vi "Parse State Queue++.vi"(0 "State Queue":string, 1 "Name(\"\" to use uuid)":string, 7 "Error In (no error)":errorcluster, 9 "Dequeue Timeout(0ms)":i32, 11 "Response Timeout(1000ms)":i32=10000) -> (4 "Remaining States":string, 6 "Current State":string, 8 "Arguments":string, 15 "From Who":string)   [LabVIEW 2014, in "JKI-State-Machine-Plus.lvlib"]
doc: "Parses the JKI State Machine state queue and returns the current state that will execute next with the associated arguments.\n\nFor instructions on how to use the JKI State Machine, examples and video tutorials, visit:\nhttp://jkisoft.com/state-machine/\n\n<B>Inputs:</B>\n <B>State Queue:</B> The entire state queue is wired to this input. This should come from the main JKI State Machine shift register.\n <B>Error In</B> The error cluster from the JKI State Machine is wired to this input. If an error occures and appears on this input, the current state output returns the \"Error Handler\" state.\n\n<B>Outputs:</B>\n <B>Remaining States:</B> Returns all the next states that should execute after the current state completes. These should be passed through the current state in the state machine. These can also be modified or augmented within the current state if necessary.\n <B>Current State:</B> Returns the current state that should execute next in the state machine. If an error is wired to the Error input then the current state output becomes \"Error Handler\".\n <B>Arguments:</B> Returns any argument(s) that may be used in the current state string. These arguments come after the \">>\" characters. <B>Note:</B> The arguments variable must not contain any unprintable characters like linefeed or carriage return.\n\n<B>State Syntax:</B>\nStateCategory: State >> Argument\nLine Terminator: Line feed\n <B>Example:</B>\nUI: Help >> About\n\nWhere \"UI\" is the state category\nWhere \"Help\" is the state\nWhere \"About\" is the argument\n <B>Other Examples:</B>\nApp Data: Initialize\nUI: Initialize\nHelp >> About\n\n<B>Commenting:</B>\nTo add a comment use \"//\" or \"#\" and all text to the right will be ignored\n <B>Commenting Example:</B>\nUI: Initialize // This initializes the UI\n# This whole line is a comment\n// Another comment line\n\nJKI State Machine™ 2018.0.7.45\nhttp://jki.net/state-machine/\nCopyright (C) 2005-2018, JKI <info@jki.net>\nALL RIGHTS RESERVED"
uses:
  JKI-State-Machine-Plus.lvlib
  _Support/_Cross JKI StateMachine State Data.ctl
  _Support/_Cross JKI StateMachine State Response.ctl
  _Support/_uuid.vi
  <vilib>/addons/_JKI Toolkits/State Machine/_JKI_lib_State_Machine.llb/Add State(s) to Queue__JKI_lib_State_Machine.vi
  Build State String with Arguments++.vi
  _Support/_JKISMQFGV.vi
  <vilib>/regexp/Match Regular Expression.xnode
panel:
  # "For instructions on how to use the JKI State Machine, examples and video tutorials, visit:\nhttp://jki.net/state-machine/\n\nJKI State Machine™\nhttp://jki.net/state-machine/\nCopyright (C) 2005-2017, JKI <info@jki.net>\nALL RIGHTS RESERVED"
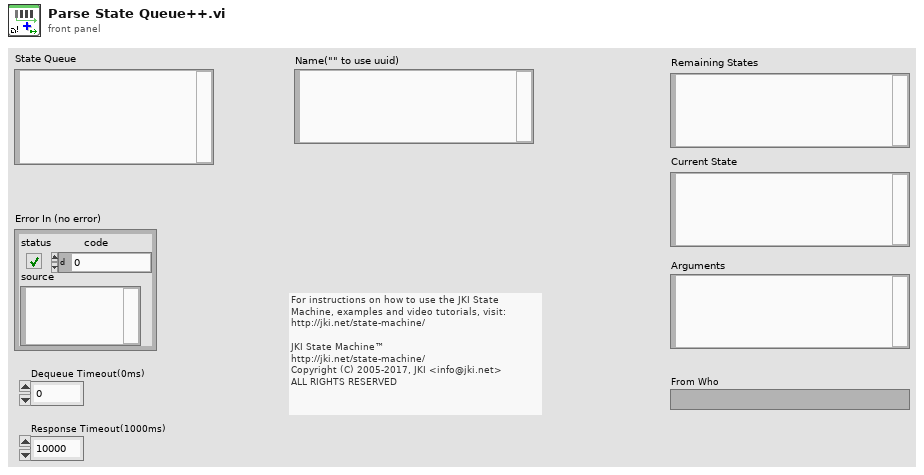
[diagram p1: front panel]
types:
  T1 = typedef "JKI-State-Machine-Plus.lvlib/_Cross JKI StateMachine State Data.ctl" = cluster{"state":string, "args":string, "source":string, "RespQ":refnum<queue>}
  T2 = typedef "JKI-State-Machine-Plus.lvlib/_Cross JKI StateMachine State Response.ctl" = cluster{"error":errorcluster}
  T3 = typedef "JKI-State-Machine-Plus.lvlib/_JKISMQ.ctl" = cluster{"Queue":refnum<queue>, "Locked Status":refnum<data-value>, "Stand Alone Mode":bool}
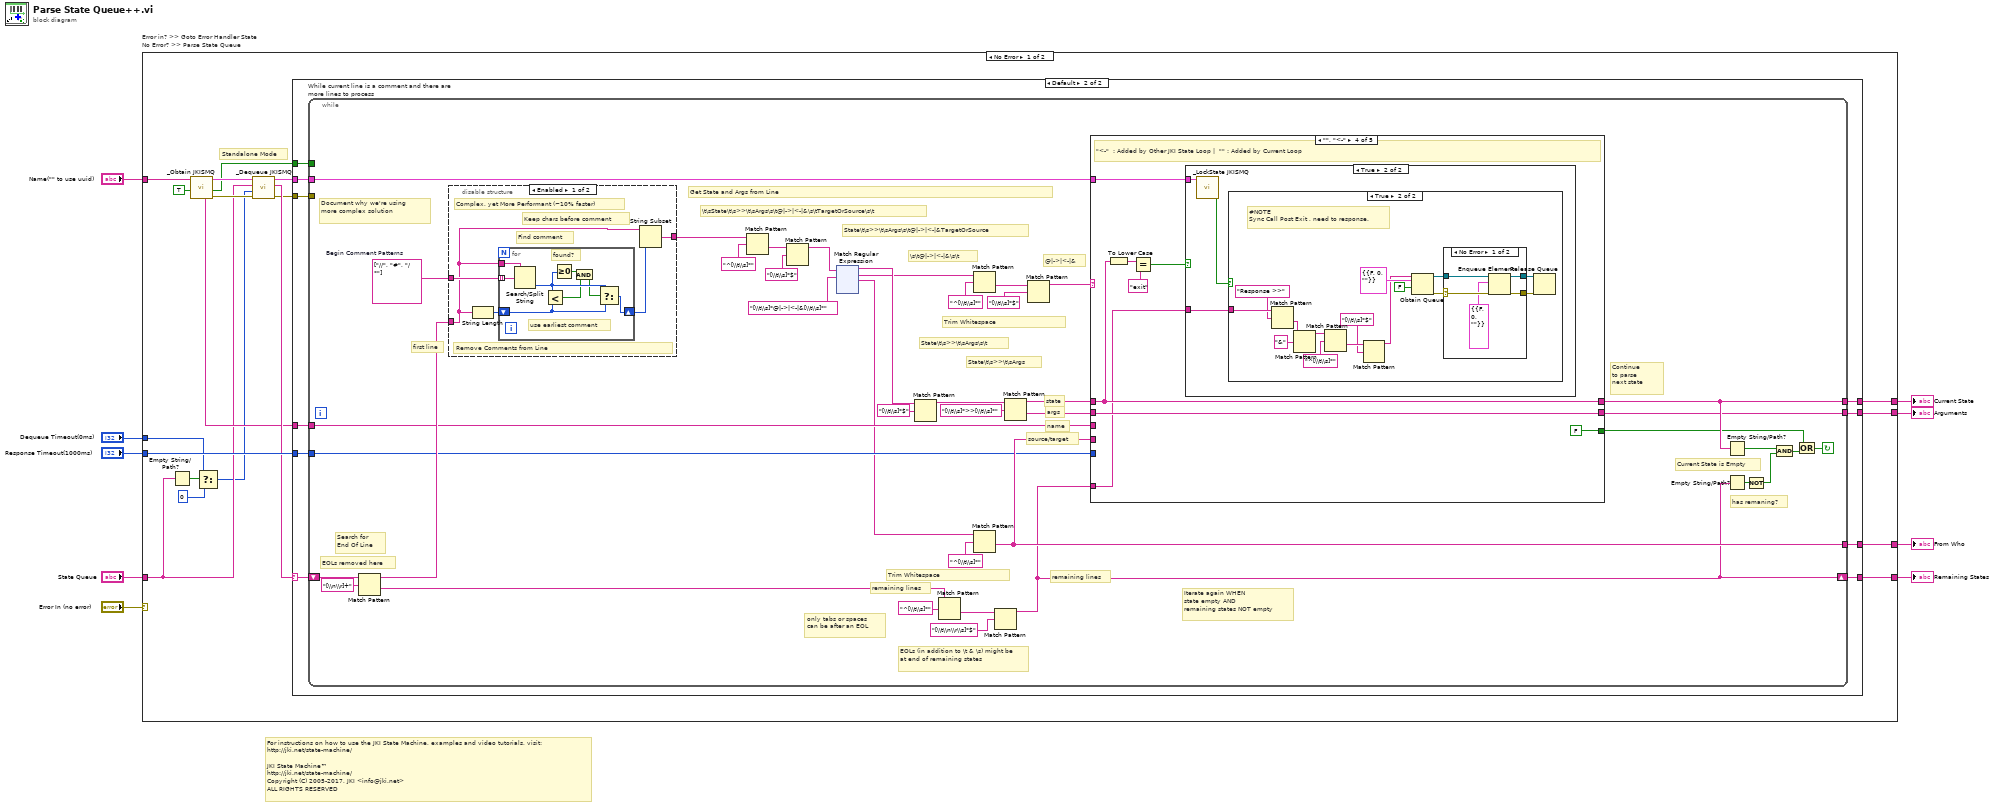
[diagram p0: block diagram]
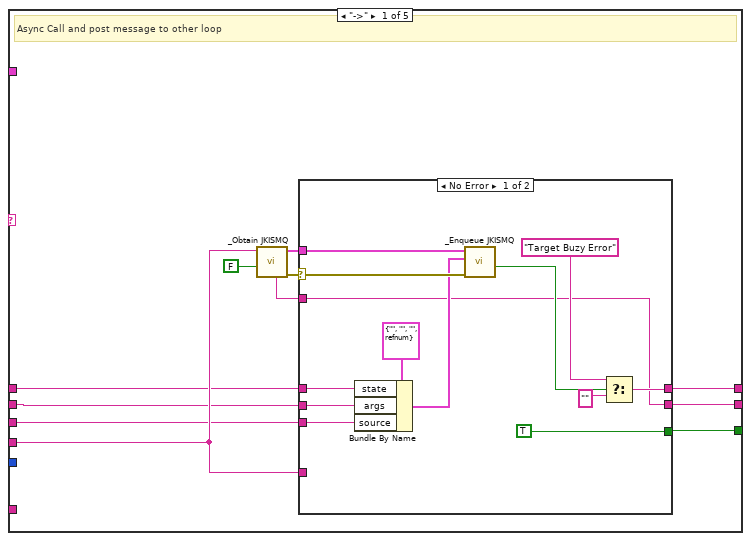
[diagram p3: hidden frame]
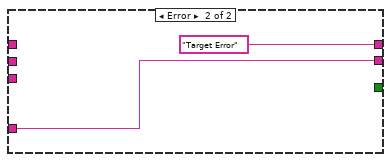
[diagram p4: hidden frame]
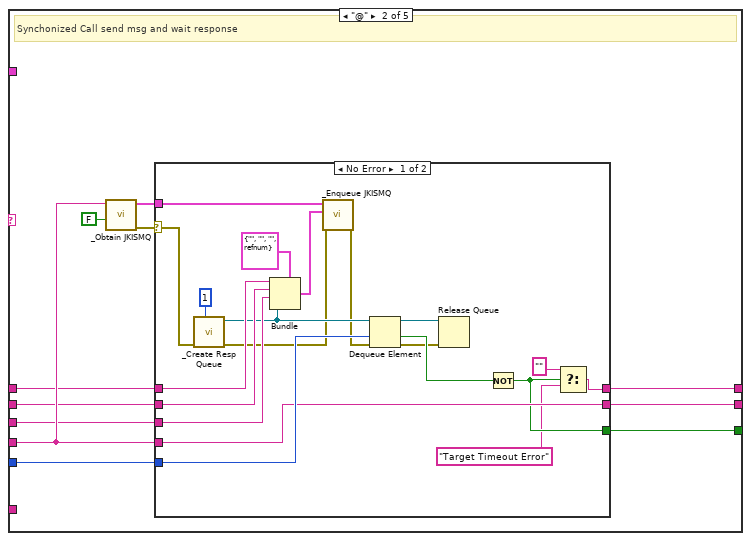
[diagram p5: hidden frame]
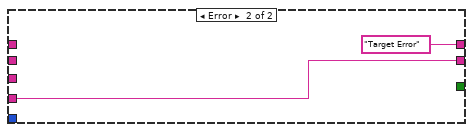
[diagram p6: hidden frame]
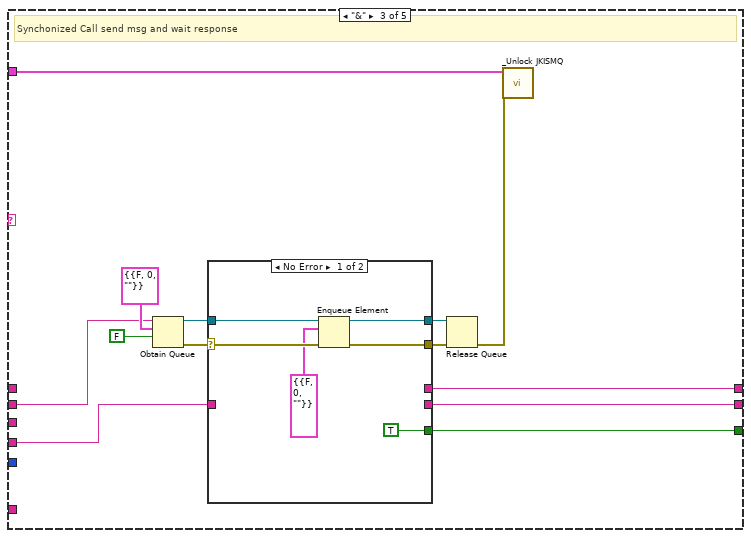
[diagram p7: hidden frame]
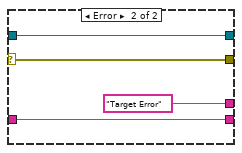
[diagram p8: hidden frame]
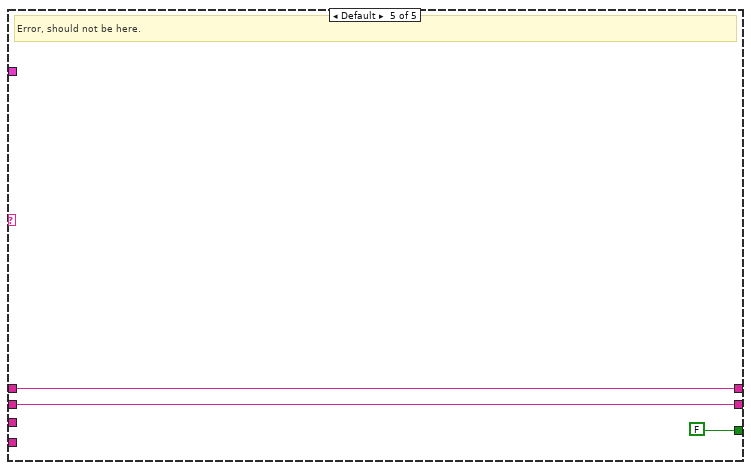
[diagram p12: hidden frame]
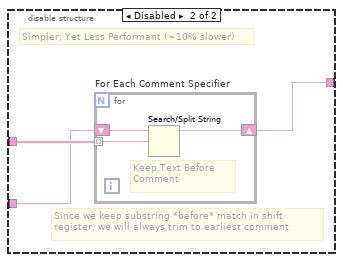
[diagram p13: hidden frame]
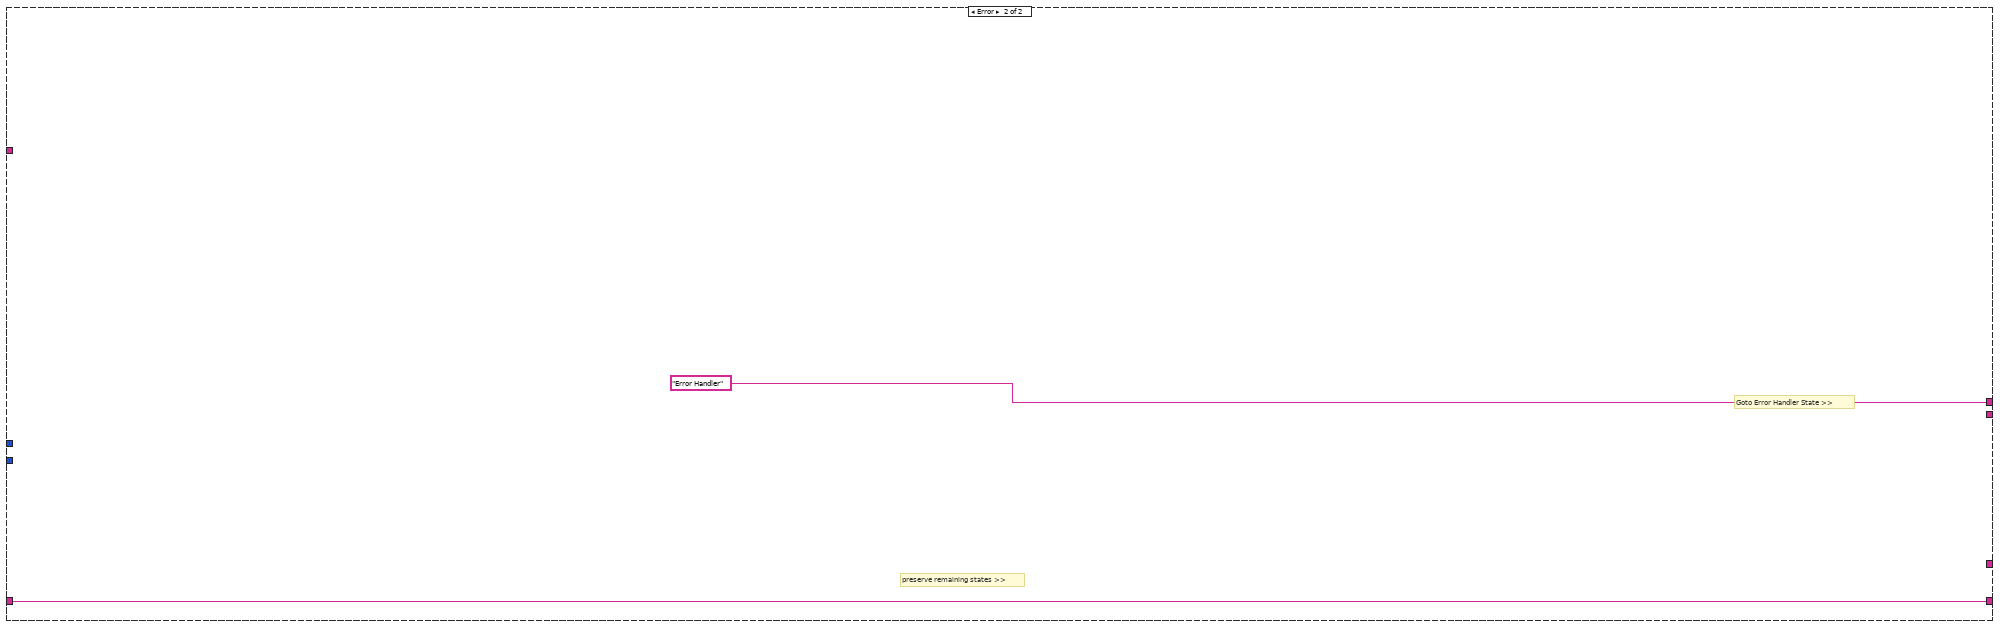
[diagram p14: hidden frame]
diagram:
  # "For instructions on how to use the JKI State Machine, examples and video tutorials, visit:\nhttp://jki.net/state-machine/\n\nJKI State Machine™\nhttp://jki.net/state-machine/\nCopyright (C) 2005-2017, JKI <info@jki.net>\nALL RIGHTS RESERVED"
  n1 = case "Error in? >> Goto Error Handler State\nNo Error? >> Parse State Queue" shown="No Error" "Error In (no error)" {
    tunnel: [w26 w331] -> w9
    tunnel: [w28 "Error Handler"] -> w7
    tunnel: [w27 _] -> w6
    tunnel: "State Queue" -> [w14 w331]
    tunnel: "Response Timeout(1000ms)" -> [w25 _]
    tunnel: "Name(\"\" to use uuid)" -> [w24 _]
    tunnel: [w23 _] -> w2
    tunnel: "Dequeue Timeout(0ms)" -> [w13 _]
    frame No Error {
      # "Standalone Mode"
      n2 = Empty String/Path?(string/path=w14) -> (empty?=w15:bool)
      n3 = call "_Obtain JKISMQ.vi"("create if not found? (T)"=TRUE, "Name(\"\" to use uuid) in"=w24) -> ("Error out"=w20:errorcluster, "Stand Alone Mode"=w10:bool, "JKISMQ"=w22:T3, "Name"=w17:string)  [unwired: 6 in]
      n4 = Select(t=w13, s=w15, f=0) -> (s? t:f=w11:i32)
      n5 = call "_Dequeue JKISMQ.vi"("Error in"=w20, "Dequeue Timeout(0ms)"=w11, "State(s) in (\"\")"=w14, "JKISMQ"=w22) -> ("Error out"=w16:errorcluster, "States Out"=w18:string, "JKISMQ"=w19:T3)  [unwired: 5 in]
      n6 = case shown="Default" w18 {
        selector: w18 -> [_ w32]
        tunnel: [_ w38] -> w28
        tunnel: [_ w37] -> w27
        tunnel: [_ w36] -> w26
        tunnel: w25 -> [_ w35]
        tunnel: [_ w34] -> w23
        tunnel: w17 -> [_ w33]
        tunnel: w19 -> [_ w31]
        tunnel: w16 -> [_ w30]
        tunnel: w10 -> [_ w29]
        frame "" {
          # "Do Nothing if Empty String"
          # "<< Wiring into the Case Selector is much more performant than using \"Empty String/Path?\" primitive"
        }
        frame Default {
          n7 = while "While current line is a comment and there are more lines to process" {
            tunnel: [w69] -> w38
            tunnel: [w68] -> w37
            shift-right: [w60] -> w36
            shift-left: w32 -> [w75]
            tunnel: w35 -> [w62]
            tunnel: w33 -> [w67]
            tunnel: [w66] -> w34
            tunnel: w31 -> [w61]
            tunnel: w30 -> [_]
            tunnel: w29 -> [_]
            stop <- w65 continue-if-true
            w74 = string[] ["//", "#", "/*"]  # Begin Comment Patterns
            # "Continue\nto parse \nnext state"
            # "source/target"
            # "name"
            # "@|->|<-|&"
            # "\\s\\t@|->|<-|&\\s\\t"
            # "Trim Whitespace"
            # "State\\t\\s>>\\t\\sArgs"
            # "State\\t\\s>>\\t\\sArgs\\s\\t"
            # "Get State and Args from Line"
            # "State\\t\\s>>\\t\\sArgs\\s\\t@|->|<-|&TargetOrSource"
            # "\\t\\sState\\t\\s>>\\t\\sArgs\\s\\t@|->|<-|&\\s\\tTargetOrSource\\s\\t"
            # "remaining lines"
            # "EOLs (in addition to \\t & \\s) might be at end of remaining states"
            # "Trim Whitespace"
            # "only tabs or spaces can be after an EOL"
            # "remaining lines"
            # "Iterate again WHEN\nstate empty AND\nremaining states NOT empty"
            # "args"
            # "state"
            # "Document why we're using more complex solution"
            # "EOLs removed here"
            # "Current State is Empty"
            # "has remaning?"
            # "first line"
            # "Search for End Of Line"
            n8 = Match Pattern(string=w75, regular expression="[\\n\\r]+") -> (before substring=w72:string, after substring=w70:string)  [unwired: 1 in, 2 out]
            n9 = disable-structure "Diagram Disable Structure" shown="Enabled" {
              disable-tunnel: w74 -> [w315 w326]
              disable-tunnel: [w314 w325] -> w73
              disable-tunnel: w72 -> [w313 w324]
              frame Enabled {
                # "Remove Comments from Line"
                # "Complex, yet More Performant (~10% faster)"
                # "Keep chars before comment"
                # "Find comment"
                n10 = String Length(string=w313) -> (length=w312:i32)
                n11 = for {
                  tunnel: w315 -> [w320] mode=indexing
                  shift-right: [w322] -> w311
                  shift-left: w312 -> [w323]
                  tunnel: w313 -> [w321]
                  # "found?"
                  # "use earliest comment"
                  n12 = Search/Split String(string=w321, search string/char (-)=w320) -> (offset of match=w319:i32)  [unwired: 1 in, 2 out]
                  n13 = Less?(x=w319, y=w323) -> (x < y?=w317:bool)
                  n14 = Greater Or Equal To 0?(x=w319) -> (x >= 0?=w318:bool)
                  n15 = And(x=w318, y=w317) -> (x .and. y?=w316:bool)
                  n16 = Select(t=w319, s=w316, f=w323) -> (s? t:f=w322:i32)
                }
                n17 = String Subset(string=w313, length (rest)=w311) -> (substring=w314:string)  [unwired: 1 in]
              }
              frame Disabled {
                # "Since we keep substring *before* match in shift register, we will always trim to earliest comment"
                # "Simpler, Yet Less Performant (~10% slower)"
                n18 = for "For Each Comment Specifier" {
                  tunnel: w326 -> [w328] mode=indexing
                  shift-right: [w327] -> w325
                  shift-left: w324 -> [w329]
                  # "Keep Text Before Comment"
                  n19 = Search/Split String(string=w329, search string/char (-)=w328) -> (substring before match=w327:string)  [unwired: 1 in, 2 out]
                }
              }
            }
            n20 = Match Pattern(string=w73, regular expression="^[\\t\\s]*") -> (after substring=w53:string)  [unwired: 1 in, 3 out]
            n21 = Match Pattern(string=w53, regular expression="[\\t\\s]*$") -> (before substring=w39:string)  [unwired: 1 in, 3 out]
            n22 = xnode "Match Regular Expression"("input string"=w39, "regular expression"="[\\t\\s]*@|->|<-|&[\\t\\s]*") -> ("before match"=w50:string, "whole match"=w47:string, "after match"=w40:string)  [unwired: 4 in, 2 out]
            n23 = Match Pattern(string=w50, regular expression="[\\t\\s]*$") -> (before substring=w49:string)  [unwired: 1 in, 3 out]
            n24 = Match Pattern(string=w70, regular expression="^[\\t\\s]*") -> (after substring=w54:string)  [unwired: 1 in, 3 out]
            n25 = Match Pattern(string=w47, regular expression="^[\\t\\s]*") -> (after substring=w43:string)  [unwired: 1 in, 3 out]
            n26 = Match Pattern(string=w40, regular expression="^[\\t\\s]*") -> (after substring=w66:string)  [unwired: 1 in, 3 out]
            n27 = Match Pattern(string=w54, regular expression="[\\t\\n\\r\\s]*$") -> (before substring=w60:string)  [unwired: 1 in, 3 out]
            n28 = Match Pattern(string=w49, regular expression="[\\t\\s]*>>[\\t\\s]*") -> (before substring=w46:string, after substring=w45:string)  [unwired: 1 in, 2 out]
            n29 = Match Pattern(string=w43, regular expression="[\\t\\s]*$") -> (before substring=w42:string)  [unwired: 1 in, 3 out]
            n30 = case shown="\"\", \"<-\"" w42 {
              tunnel: w46 -> [w82 w107 _ w166 w196]
              tunnel: w45 -> [w81 w106 w140 w168 w195]
              tunnel: [w88 w113 w149 w166 w196] -> w69
              tunnel: [w87 w112 w148 w168 w195] -> w68
              tunnel: w67 -> [w80 w105 _ _ _]
              tunnel: w66 -> [w85 w111 w141 _ _]
              tunnel: [w89 w114 w150 FALSE FALSE] -> w63
              tunnel: w62 -> [_ w115 _ _ _]
              tunnel: w61 -> [_ _ w139 w161 _]
              tunnel: w60 -> [_ _ _ w163 _]
              frame "->" {
                # "Async Call and post message to other loop"
                n31 = call "_Obtain JKISMQ.vi"("create if not found? (T)"=FALSE, "Name(\"\" to use uuid) in"=w85) -> ("Error out"=w83:errorcluster, "JKISMQ"=w84:T3, "Name"=w79:string)  [unwired: 6 in, 1 out]
                n32 = case shown="No Error" w83 {
                  selector: w83 -> [w101 _]
                  tunnel: w84 -> [w102 _]
                  tunnel: [TRUE _] -> w89
                  tunnel: [w91 "Target Error" ("before match")] -> w88
                  tunnel: [w90 w103] -> w87
                  tunnel: w85 -> [_ w103]
                  tunnel: w82 -> [w98 _]
                  tunnel: w81 -> [w97 _]
                  tunnel: w80 -> [w96 _]
                  tunnel: w79 -> [w90 _]
                  frame No Error {
                    n33 = Bundle By Name(cluster=T1 {"state"="", "args"="", "source"="", "RespQ"=refnum} ("Cross JKI State Machine State"), "state"=w98, "args"=w97, "source"=w96) -> (w95:T1)
                    n34 = call "_Enqueue JKISMQ.vi"("Error in"=w101, "Data"=w95, "JKISMQ"=w102) -> ("Target Buzy Error"=w92:bool)  [unwired: 6 in, 2 out]
                    n35 = Select(t="Target Buzy Error" ("f"), s=w92, f="" ("before match")) -> (s? t:f=w91:string)
                  }
                  frame Error {
                  }
                }
              }
              frame "@" {
                # "Synchonized Call send msg and wait response"
                n36 = call "_Obtain JKISMQ.vi"("create if not found? (T)"=FALSE, "Name(\"\" to use uuid) in"=w111) -> ("Error out"=w109:errorcluster, "JKISMQ"=w110:T3)  [unwired: 6 in, 2 out]
                n37 = case shown="No Error" w109 {
                  selector: w109 -> [w120 _]
                  tunnel: w115 -> [w134 _]
                  tunnel: w110 -> [w135 _]
                  tunnel: [w130 _] -> w114
                  tunnel: [w133 "Target Error" ("before match")] -> w113
                  tunnel: [w132 w136] -> w112
                  tunnel: w111 -> [w132 w136]
                  tunnel: w107 -> [w126 _]
                  tunnel: w106 -> [w125 _]
                  tunnel: w105 -> [w124 _]
                  frame No Error {
                    n38 = call "_Create Resp Queue.vi"("max queue size (-1, unlimited)"=1, "error in (no error)"=w120) -> ("error out"=w116:errorcluster, "queue out"=w121:refnum<queue>)  [unwired: 7 in, 1 out]
                    n39 = Bundle(cluster=T1 {"state"="", "args"="", "source"="", "RespQ"=refnum} ("Cross JKI State Machine State"), "state"=w126, "args"=w125, "source"=w124, "RespQ"=w121) -> (w122:T1)
                    n40 = call "_Enqueue JKISMQ.vi"("Error in"=w116, "Data"=w122, "JKISMQ"=w135) -> ("Error out"=w117:errorcluster)  [unwired: 6 in, 2 out]
                    n41 = Dequeue Element(queue=w121, timeout in ms (-1)=w134, error in (no error)=w117) -> (queue out=w119:refnum<queue>, timed out?=w131:bool, error out=w118:errorcluster)  [unwired: 1 out]
                    n42 = Release Queue(queue=w119, error in (no error)=w118) -> ()  [unwired: 1 in, 3 out]
                    n43 = Not(x=w131) -> (.not. x?=w130:bool)
                    n44 = Select(t="" ("f"), s=w130, f="Target Timeout Error" ("before match")) -> (s? t:f=w133:string)
                  }
                  frame Error {
                  }
                }
              }
              frame "&" {
                # "Synchonized Call send msg and wait response"
                n45 = Obtain Queue(name (unnamed)=w140, element data type=T2 {"error"={"status"=FALSE, "code"=0, "source"=""}} ("Cross JKI State Machine Response"), create if not found? (T)=FALSE) -> (queue out=w145:refnum<queue>, error out=w144:errorcluster)  [unwired: 2 in, 1 out]
                n46 = case shown="No Error" w144 {
                  selector: w144 -> [w154 w158]
                  tunnel: [TRUE _] -> w150
                  tunnel: [_ "Target Error" ("before match")] -> w149
                  tunnel: [_ w157] -> w148
                  tunnel: w145 -> [w156 w159]
                  tunnel: [w155 w159] -> w147
                  tunnel: [w153 w158] -> w146
                  tunnel: w141 -> [_ w157]
                  frame No Error {
                    n47 = Enqueue Element(queue=w156, element=T2 {"error"={"status"=FALSE, "code"=0, "source"=""}}, error in (no error)=w154) -> (queue out=w155:refnum<queue>, error out=w153:errorcluster)  [unwired: 1 in, 1 out]
                  }
                  frame Error {
                  }
                }
                n48 = Release Queue(queue=w147, error in (no error)=w146) -> (error out=w138:errorcluster)  [unwired: 1 in, 2 out]
                n49 = call "_Unlock JKISMQ.vi"("Error in"=w138, "JKISMQ"=w139) -> ()  [unwired: 8 in, 2 out]
              }
              frame "", "<-" {
                # "\"<-\"  : Added by Other JKI State Loop |  \"\" : Added by Current Loop"
                n50 = To Lower Case(string=w166) -> (all lower case string=w165:string)
                n51 = Equal?(x=w165, y="exit") -> (x = y?=w162:bool)
                n52 = case shown="True" w162 {
                  tunnel: w163 -> [_ w171]
                  tunnel: w161 -> [_ w170]
                  frame False {
                  }
                  frame True {
                    n53 = call "_LockState JKISMQ.vi"("JKISMQ"=w170) -> ("lock"=w169:bool)  [unwired: 8 in, 2 out]
                    n54 = case shown="True" w169 {
                      tunnel: w171 -> [_ w180]
                      frame False {
                      }
                      frame True {
                        # "#NOTE\nSync Call Post Exit , need to response."
                        n55 = Match Pattern(string=w180, regular expression="Response >>") -> (after substring=w177:string)  [unwired: 1 in, 3 out]
                        n56 = Match Pattern(string=w177, regular expression="&") -> (before substring=w173:string)  [unwired: 1 in, 3 out]
                        n57 = Match Pattern(string=w173, regular expression="^[\\t\\s]*") -> (after substring=w176:string)  [unwired: 1 in, 3 out]
                        n58 = Match Pattern(string=w176, regular expression="[\\t\\s]*$") -> (before substring=w172:string)  [unwired: 1 in, 3 out]
                        n59 = Obtain Queue(name (unnamed)=w172, element data type=T2 {"error"={"status"=FALSE, "code"=0, "source"=""}} ("Cross JKI State Machine Response"), create if not found? (T)=FALSE) -> (queue out=w185:refnum<queue>, error out=w186:errorcluster)  [unwired: 2 in, 1 out]
                        n60 = case shown="No Error" w186 {
                          selector: w186 -> [w189 w192]
                          tunnel: w185 -> [w191 w193]
                          tunnel: [w190 w193] -> w183
                          tunnel: [w188 w192] -> w184
                          frame No Error {
                            n61 = Enqueue Element(queue=w191, element=T2 {"error"={"status"=FALSE, "code"=0, "source"=""}}, error in (no error)=w189) -> (queue out=w190:refnum<queue>, error out=w188:errorcluster)  [unwired: 1 in, 1 out]
                          }
                          frame Error {
                          }
                        }
                        n62 = Release Queue(queue=w183, error in (no error)=w184) -> ()  [unwired: 1 in, 3 out]
                      }
                    }
                  }
                }
              }
              frame Default {
                # "Error, should not be here."
              }
            }
            n63 = Empty String/Path?(string/path=w69) -> (empty?=w78:bool)
            n64 = Empty String/Path?(string/path=w60) -> (empty?=w77:bool)
            n65 = Not(x=w77) -> (.not. x?=w71:bool)
            n66 = And(x=w78, y=w71) -> (x .and. y?=w64:bool)
            n67 = Or(x=w63, y=w64) -> (x .or. y?=w65:bool)
          }
        }
      }
    }
    frame Error {
      # "Goto Error Handler State >>"
      # "preserve remaining states >>"
    }
  }
  "Remaining States" <- w9
  "Arguments" <- w6
  "Current State" <- w7
  "From Who" <- w2
